vi "Allan Variance SUBVI.vi"(0 "data in":dbl[][](array[numeric]), 3 "amount":u32=100, 7 "error in (no error)":errorcluster) -> (8 "AccX - Allan Variance":cluster{i32, "Numeric":dbl, "Numeric":dbl}[](graph), 9 "AccX":T1(array[cluster]), 10 "AccY - Allan Variance":cluster{i32, "Numeric":dbl, "Numeric":dbl}[](graph), 11 "AccY":T1(array[cluster]), 12 "AccZ - Allan Variance":cluster{i32, "Numeric":dbl, "Numeric":dbl}[](graph), 13 "AccZ":T1(array[cluster]), 14 "GyrX - Allan Variance":cluster{i32, "Numeric":dbl, "Numeric":dbl}[](graph), 15 "GyrX":T1(array[cluster]), 16 "GyrY - Allan Variance":cluster{i32, "Numeric":dbl, "Numeric":dbl}[](graph), 17 "GyrY":T1(array[cluster]), 18 "GyrZ - Allan Variance":cluster{i32, "Numeric":dbl, "Numeric":dbl}[](graph), 19 "GyrZ":T1(array[cluster]), 21 "MagX - Allan Variance":cluster{i32, "Numeric":dbl, "Numeric":dbl}[](graph), 22 "MagY - Allan Variance":cluster{i32, "Numeric":dbl, "Numeric":dbl}[](graph), 23 "MagZ - Allan Variance":cluster{i32, "Numeric":dbl, "Numeric":dbl}[](graph), 24 "MagZ":T1(array[cluster]), 25 "MagY":T1(array[cluster]), 26 "MagX":T1(array[cluster]), 27 "error out":errorcluster)   [LabVIEW 2021, in "IMU Processing.lvlib"]
uses:
  IMU Processing.lvlib
  ErrorModellingLibrary/VIs/Allan Variance Chart NO.vi
  ErrorModellingLibrary/ErrorModellingLibrary.lvlib
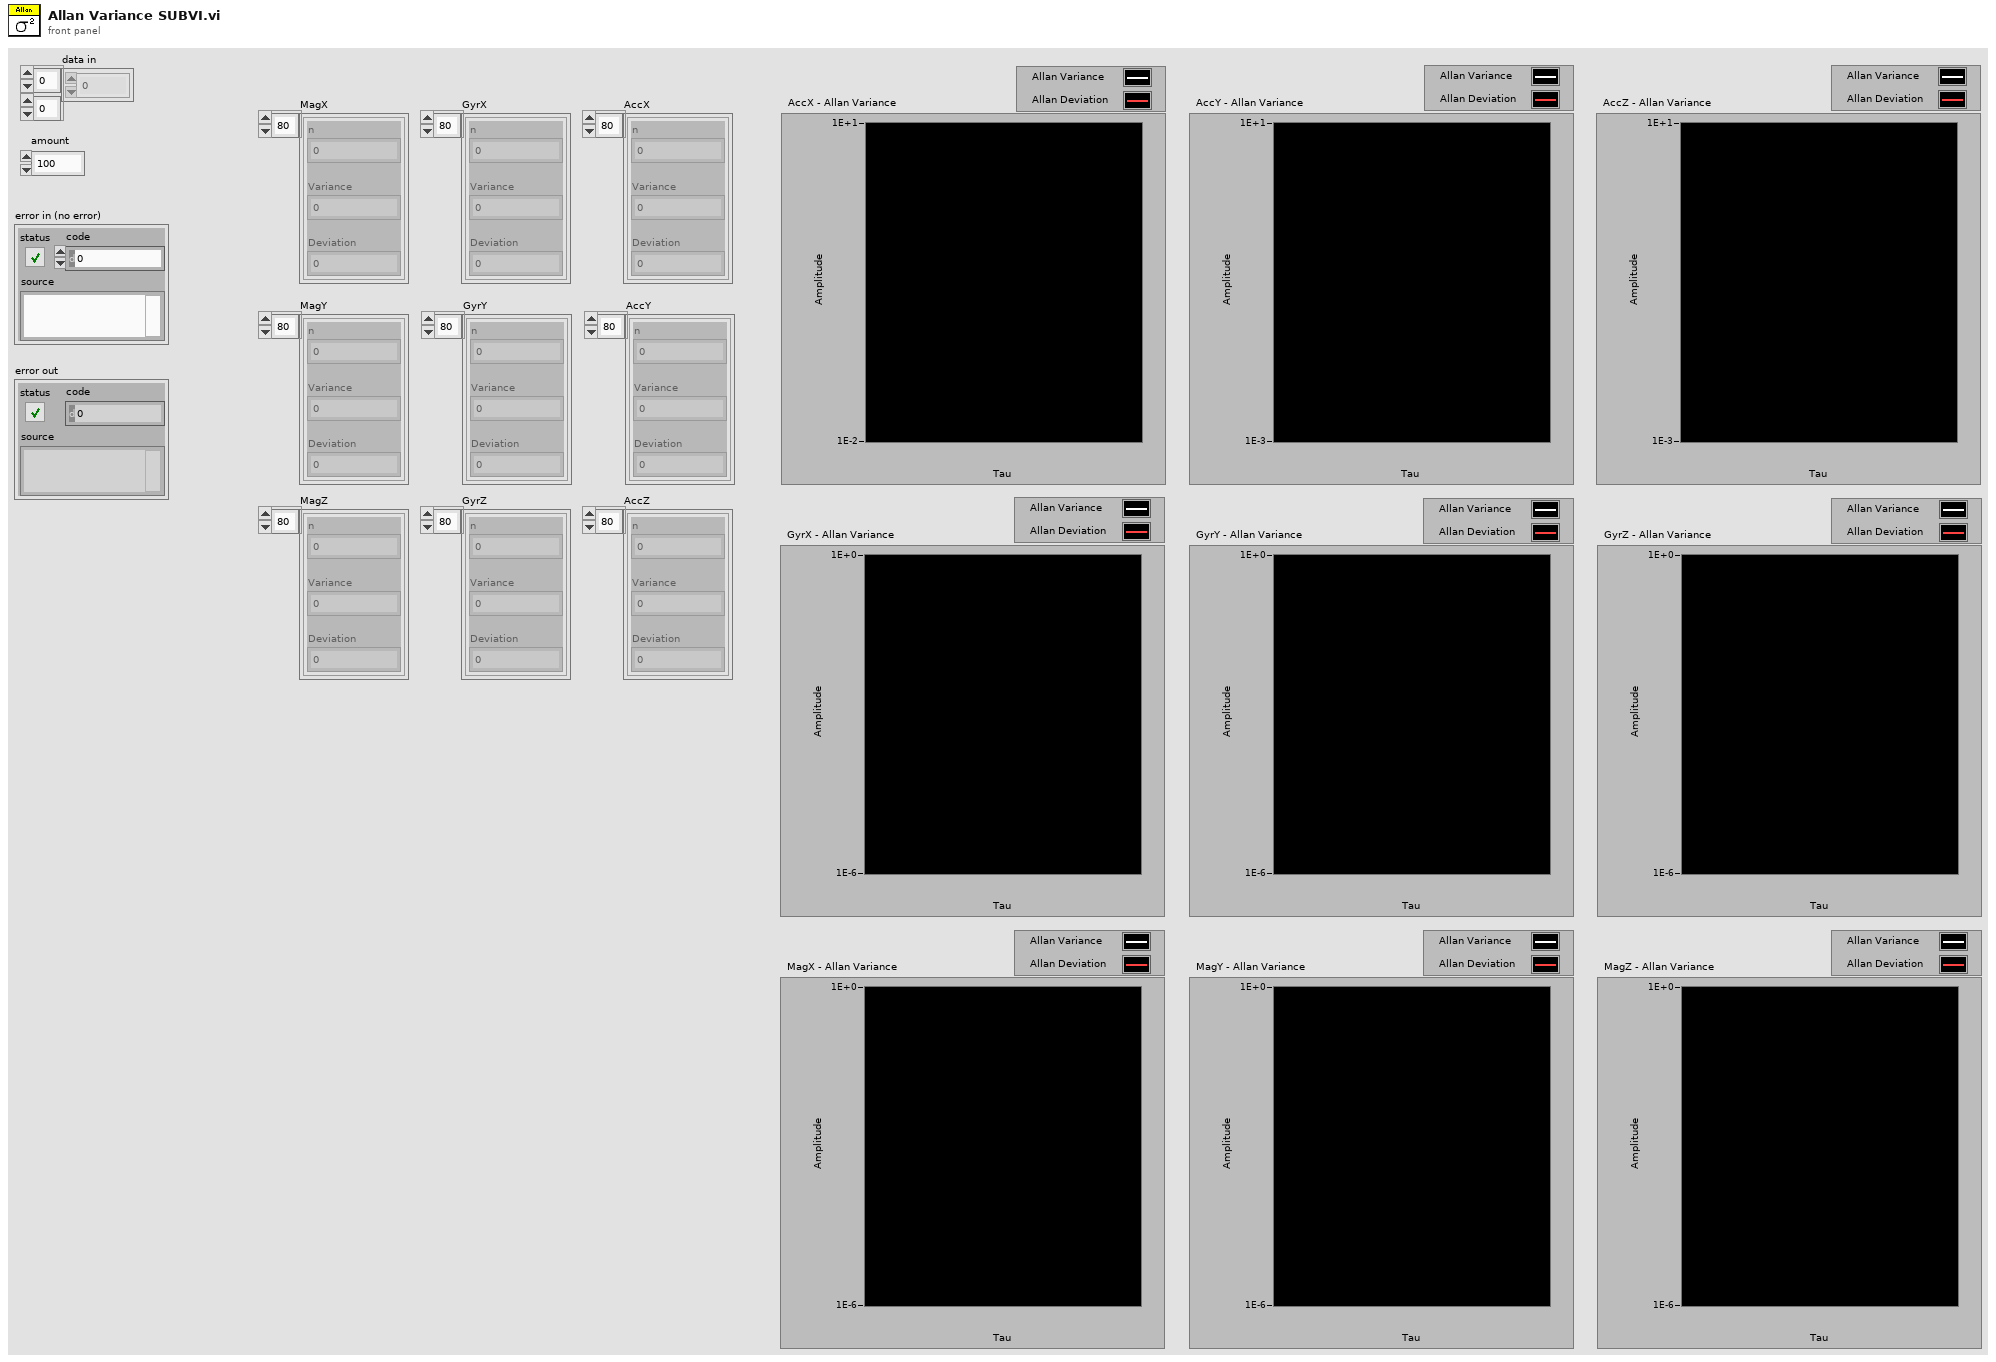
[diagram p1: front panel]
types:
  T1 = cluster{"n":i32, "Variance":dbl, "Deviation":dbl}[]
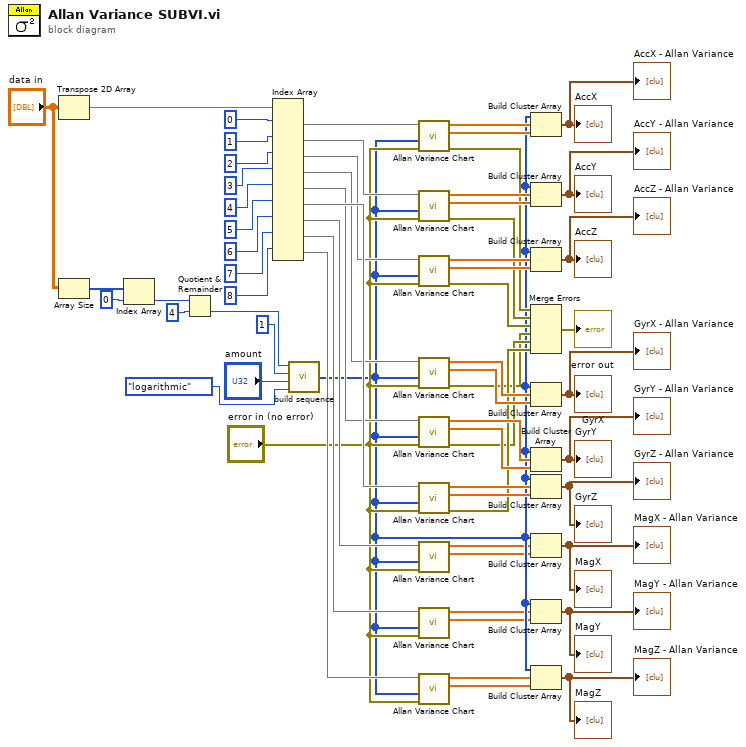
[diagram p0: block diagram]
diagram:
  n1 = Transpose 2D Array(2D array="data in") -> (transposed array=w18:dbl[][])
  n2 = Array Size(array="data in") -> (size(s)=w38:i32[])
  n3 = Index Array(array=w38, index=0) -> (element=w40:i32)
  n4 = Quotient & Remainder(x=w40, y=4) -> (floor(x/y)=w45:i32)  [unwired: 1 out]
  n5 = Index Array(array=w18, index (row) #1=0 ("index (row)"), index (row) #2=1 ("index (row)"), index (row) #3=2 ("index (row)"), index (row) #4=3 ("index (row)"), index (row) #5=4 ("index (row)"), index (row) #6=5 ("index (row)"), index (row) #7=6 ("index (row)"), index (row) #8=7 ("index (row)"), index (row) #9=8 ("index (row)")) -> (element #1=w25:dbl[], element #2=w27:dbl[], element #3=w28:dbl[], element #4=w29:dbl[], element #5=w30:dbl[], element #6=w31:dbl[], element #7=w14:dbl[], element #8=w13:dbl[], element #9=w12:dbl[])  [unwired: 9 in]
  n6 = call "build sequence.vi"("Enum"=enum16{"logarithmic", "linear"}."logarithmic", "amount"="amount", "min"=u32 1, "max"=w45) -> ("Array - Numeric"=w10:i32[])
  n7 = call-poly "Allan Variance Chart.vi"("error in (no error)"="error in (no error)", "nArray"=w10, "inputdata"=w25) -> ("error out"=w26:errorcluster, "Allan Deviation"=w47:dbl[], "Allan Variance"=w46:dbl[])  [unwired: 6 in]
  n8 = call-poly "Allan Variance Chart.vi"("error in (no error)"="error in (no error)", "nArray"=w10, "inputdata"=w27) -> ("error out"=w32:errorcluster, "Allan Deviation"=w50:dbl[], "Allan Variance"=w49:dbl[])  [unwired: 6 in]
  n9 = call-poly "Allan Variance Chart.vi"("error in (no error)"="error in (no error)", "nArray"=w10, "inputdata"=w28) -> ("error out"=w33:errorcluster, "Allan Deviation"=w52:dbl[], "Allan Variance"=w51:dbl[])  [unwired: 6 in]
  n10 = call-poly "Allan Variance Chart.vi"("error in (no error)"="error in (no error)", "nArray"=w10, "inputdata"=w29) -> ("error out"=w34:errorcluster, "Allan Deviation"=w54:dbl[], "Allan Variance"=w53:dbl[])  [unwired: 6 in]
  n11 = call-poly "Allan Variance Chart.vi"("error in (no error)"="error in (no error)", "nArray"=w10, "inputdata"=w30) -> ("error out"=w35:errorcluster, "Allan Deviation"=w56:dbl[], "Allan Variance"=w55:dbl[])  [unwired: 6 in]
  n12 = call-poly "Allan Variance Chart.vi"("error in (no error)"="error in (no error)", "nArray"=w10, "inputdata"=w31) -> ("error out"=w36:errorcluster, "Allan Deviation"=w58:dbl[], "Allan Variance"=w57:dbl[])  [unwired: 6 in]
  n13 = call-poly "Allan Variance Chart.vi"("error in (no error)"="error in (no error)", "nArray"=w10, "inputdata"=w14) -> ("Allan Deviation"=w8:dbl[], "Allan Variance"=w9:dbl[])  [unwired: 6 in, 1 out]
  n14 = call-poly "Allan Variance Chart.vi"("error in (no error)"="error in (no error)", "nArray"=w10, "inputdata"=w13) -> ("Allan Deviation"=w6:dbl[], "Allan Variance"=w7:dbl[])  [unwired: 6 in, 1 out]
  n15 = call-poly "Allan Variance Chart.vi"("error in (no error)"="error in (no error)", "nArray"=w10, "inputdata"=w12) -> ("Allan Deviation"=w4:dbl[], "Allan Variance"=w5:dbl[])  [unwired: 6 in, 1 out]
  n16 = Build Cluster Array(w10, w46, w47) -> (→"AccX - Allan Variance" →"AccX":cluster{i32, "Numeric":dbl, "Numeric":dbl}[])
  n17 = Build Cluster Array(w10, w49, w50) -> (→"AccY - Allan Variance" →"AccY":cluster{i32, "Numeric":dbl, "Numeric":dbl}[])
  n18 = Build Cluster Array(w10, w51, w52) -> (→"AccZ - Allan Variance" →"AccZ":cluster{i32, "Numeric":dbl, "Numeric":dbl}[])
  n19 = Merge Errors(w26, w32, w33, w34, w35, w36) -> (→"error out":errorcluster)
  n20 = Build Cluster Array(w10, w53, w54) -> (→"GyrX - Allan Variance" →"GyrX":cluster{i32, "Numeric":dbl, "Numeric":dbl}[])
  n21 = Build Cluster Array(w10, w55, w56) -> (→"GyrY - Allan Variance" →"GyrY":cluster{i32, "Numeric":dbl, "Numeric":dbl}[])
  n22 = Build Cluster Array(w10, w57, w58) -> (→"GyrZ - Allan Variance" →"GyrZ":cluster{i32, "Numeric":dbl, "Numeric":dbl}[])
  n23 = Build Cluster Array(w10, w9, w8) -> (→"MagX - Allan Variance" →"MagX":cluster{i32, "Numeric":dbl, "Numeric":dbl}[])
  n24 = Build Cluster Array(w10, w7, w6) -> (→"MagY - Allan Variance" →"MagY":cluster{i32, "Numeric":dbl, "Numeric":dbl}[])
  n25 = Build Cluster Array(w10, w5, w4) -> (→"MagZ - Allan Variance" →"MagZ":cluster{i32, "Numeric":dbl, "Numeric":dbl}[])
